vi "system_logic.vi"(2 "Lower Threshold":dbl, 3 "Upper Threshold":dbl, 4 "VISA Name in":refnum<visa-resource-name>, 5 "Value":dbl) -> (0 "Action":u16(ring)=2 items=["Infuse", "Withdraw", "No Action", "Logc Error"], 1 "VISA Name out":refnum<visa-resource-name>)   [LabVIEW 2019]
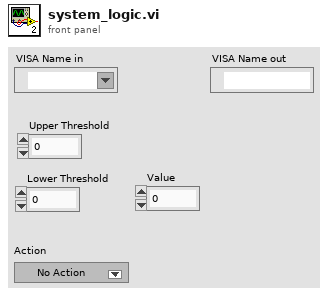
[diagram p1: front panel]
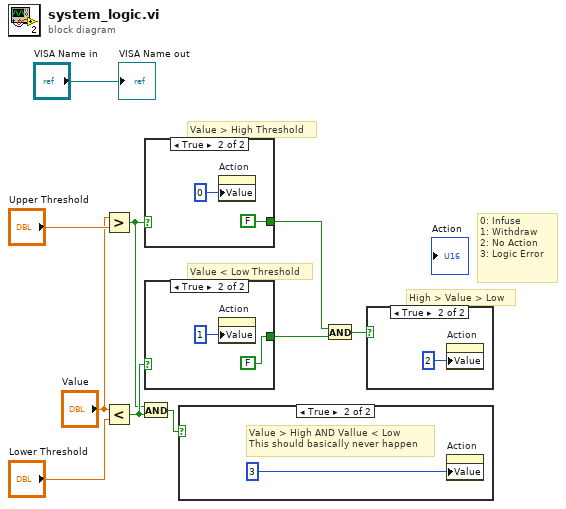
[diagram p0: block diagram]
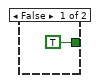
[diagram p4: hidden frame]
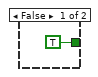
[diagram p5: hidden frame]
diagram:
  # "0: Infuse\n1: Withdraw\n2: No Action \n3: Logic Error"
  # "High > Value > Low"
  # "Value > High Threshold"
  # "Value < Low Threshold"
  n1 = Greater?(x="Value", y="Upper Threshold") -> (0:w7:bool)
  n2 = Less?(x="Value", y="Lower Threshold") -> (x < y?=w8:bool)
  n3 = And(x=w7, y=w8) -> (x .and. y?=w1:bool)
  n4 = case shown="True" w7 {
    tunnel: [TRUE FALSE] -> w9
    frame False {
    }
    frame True {
      n5 = property on="Action" class="Ring (strict)"("Value"=0) -> ()  [unwired: 2 in, 2 out]
    }
  }
  n6 = case shown="True" w8 {
    tunnel: [TRUE FALSE] -> w10
    frame False {
    }
    frame True {
      n7 = property on="Action" class="Ring (strict)"("Value"=1) -> ()  [unwired: 2 in, 2 out]
    }
  }
  n8 = case shown="True" w1 {
    frame False {
    }
    frame True {
      # "Value > High AND Vallue < Low\nThis should basically never happen"
      n9 = property on="Action" class="Ring (strict)"("Value"=3) -> ()  [unwired: 2 in, 2 out]
    }
  }
  n10 = And(x=w9, y=w10) -> (x .and. y?=w4:bool)
  n11 = case shown="True" w4 {
    frame False {
    }
    frame True {
      n12 = property on="Action" class="Ring (strict)"("Value"=2) -> ()  [unwired: 2 in, 2 out]
    }
  }
  "VISA Name out" <- "VISA Name in"
